vi "WriteTestDescription.vi"(8 "error in (no error)":errorcluster, 10 "Test Description":string="2. Ruido Intrínseco. IEC 61672-3: 2006 Cláusula 10", 11 "Prueba in":refnum<class "Prueba.lvclass">) -> (0 "error out":errorcluster, 3 "Prueba out":refnum<class "Prueba.lvclass">)   [LabVIEW 2019, in "Prueba.lvclass"]
uses:
  Prueba.lvclass
  Prueba.lvclass/Prueba.ctl
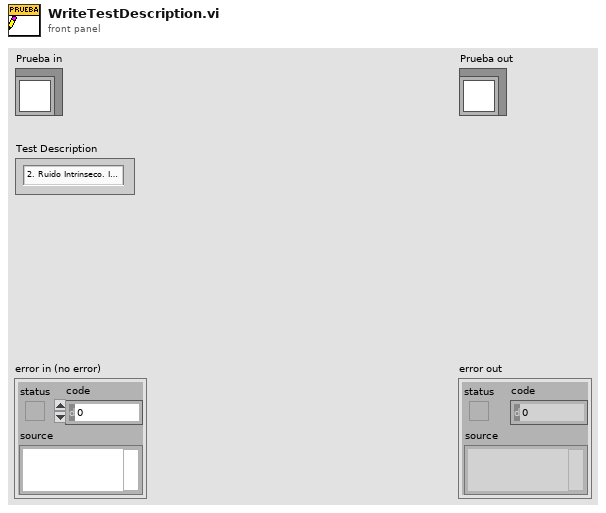
[diagram p1: front panel]
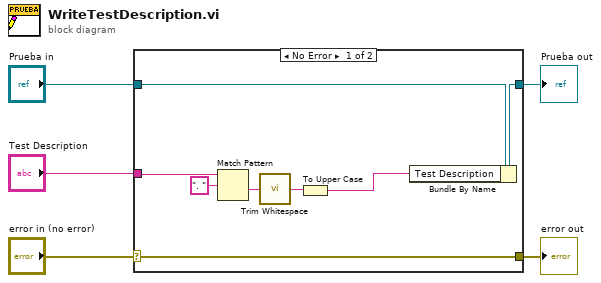
[diagram p0: block diagram]
diagram:
  n1 = case shown="No Error" "error in (no error)" {
    selector: "error in (no error)" -> [w13 w14]
    tunnel: [w13 w14] -> w4
    tunnel: [w11 w15] -> w2
    tunnel: "Prueba in" -> [w12 w15]
    tunnel: "Test Description" -> [w7 _]
    frame No Error {
      n2 = Match Pattern(string=w7, regular expression=". ") -> (after substring=w9:string)  [unwired: 1 in, 3 out]
      n3 = call <vilib>:"Trim Whitespace.vi"("string"=w9) -> ("trimmed string"=w8:string)  [unwired: 1 in]
      n4 = To Upper Case(1:w8) -> (0:w6:string)
      n5 = Bundle By Name(cluster=w12, "Test Description"=w6) -> (w11:refnum<class "Prueba.lvclass">)
    }
    frame Error {
    }
  }
  "error out" <- w4
  "Prueba out" <- w2
